vi "Single Command with parameters.vi"(8 "error in (no error)":errorcluster, 9 "Variant (simple type, or Cluster/Array)":variant, 10 "SQL (Single Command)":string, 11 "PQ Connection in":refnum<class "PQ Connection.lvclass">) -> (0 "error out":errorcluster, 1 "First Result with Rows returned":refnum<class "PQ Result.lvclass">, 2 "Number of Rows":i32, 3 "PQ Connection out":refnum<class "PQ Connection.lvclass">)   [LabVIEW 2013, in "PQ Connection.lvclass"]
uses:
  PQ Connection.lvclass
  Result/PQ Result.lvclass
  <userlib>/_OpenG.lib/lvdata/lvdata.llb/Get TDEnum from TD__ogtk.vi
  1. Sources/Lib/Lib.llb/Variant to Header Info__ogtk.vi
  Cluster to Array (recursive).vi
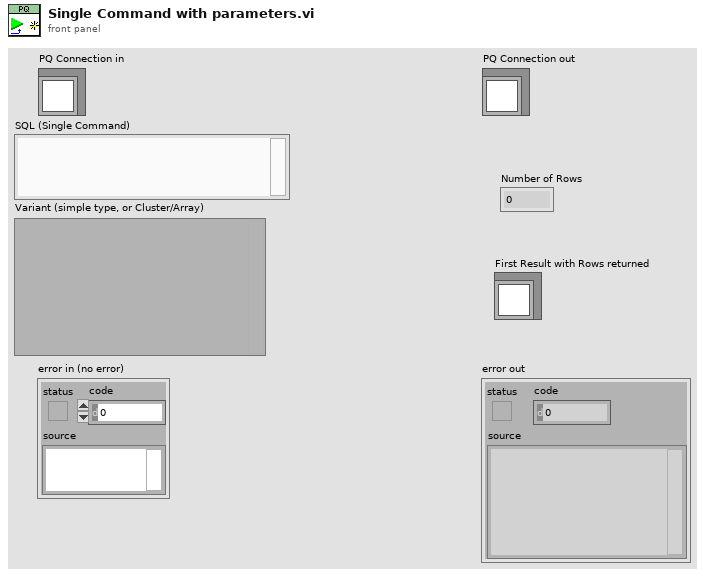
[diagram p1: front panel]
types:
  T1 = enum8{"Invalid Type", "Void", "I8", "I16", "I32", "I64", "U8", "U16", "U32", "U64", "Single Float", "Double Float", "Extended Float", "Single Complex", "Double Complex", "Extended Complex", "Enum U8", "Enum U16", "Enum U32", "Enum U64", "Single Float With Unit", "Double Float With Unit", "Extended Float With Unit", "Single Complex with Unit", "Double Complex with Unit", "Extended Complex with Unit", "Boolean", "String", "Path", "Picture", "Tag", "Array", "Cluster", "Variant", "LV Variant", "Waveform", "Timestamp", "Digital Waveform", "Digital Data", "ExpressData", "Refnum", "External Data", "VI", "Poly VI", "LabVIEW Class Instance", "Fixed Point"}[]
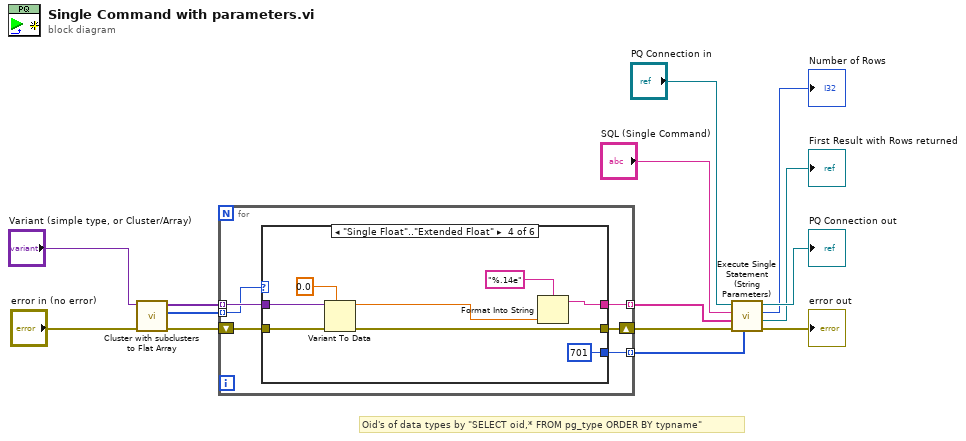
[diagram p0: block diagram]
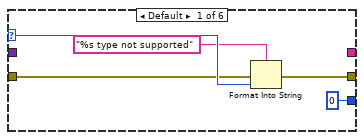
[diagram p2: hidden frame]
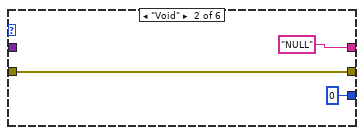
[diagram p3: hidden frame]
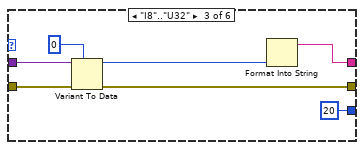
[diagram p4: hidden frame]
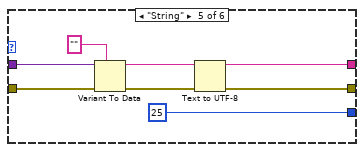
[diagram p5: hidden frame]
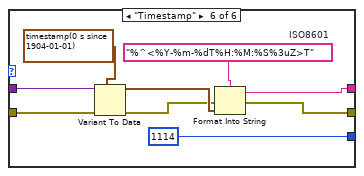
[diagram p6: hidden frame]
diagram:
  # "Oid's of data types by \"SELECT oid,* FROM pg_type ORDER BY typname\""
  n1 = call "Cluster with subclusters to Flat Array.vi"("error in (no error)"="error in (no error)", "Variant"="Variant (simple type, or Cluster/Array)") -> ("error out"=w13:errorcluster, "Types"=w1:T1, "Array of items"=w14:variant[])  [unwired: 7 in]
  n2 = for {
    tunnel: w14 -> [w20] mode=indexing
    tunnel: [w19] -> w7 mode=indexing
    shift-right: [w18] -> w8
    shift-left: w13 -> [w15]
    tunnel: [w17] -> w2 mode=indexing
    tunnel: w1 -> [w16] mode=indexing
    n3 = case shown="\"Single Float\"..\"Extended Float\"" w16 {
      selector: w16 -> [w25 _ _ _ _ _]
      tunnel: w20 -> [_ _ w35 w43 w51 w60]
      tunnel: [_ "NULL" w32 w40 w46 w52] -> w19
      tunnel: w15 -> [w23 w27 w31 w38 w49 w59]
      tunnel: [w22 w27 w30 w37 w44 w53] -> w18
      tunnel: [0 0 20 701 25 1114] -> w17
      frame Default {
        n4 = Format Into String(format string="%s type not supported", error in=w23, w25) -> (error out=w22:errorcluster)  [unwired: 1 in, 1 out]
      }
      frame "Void" {
      }
      frame "I8".."U32" {
        n5 = Variant To Data(error in=w31, type=i64 0, Variant=w35) -> (data=w33:i64, error out=w30:errorcluster)
        n6 = Format Into String(w33) -> (resulting string=w32:string)  [unwired: 3 in, 1 out]
      }
      frame "Single Float".."Extended Float" {
        n7 = Variant To Data(error in=w38, type=0.0, Variant=w43) -> (data=w41:dbl, error out=w37:errorcluster)
        n8 = Format Into String(format string="%.14e", w41) -> (resulting string=w40:string)  [unwired: 2 in, 1 out]
      }
      frame "String" {
        n9 = Variant To Data(error in=w49, type="", Variant=w51) -> (data=w47:string, error out=w45:errorcluster)
        n10 = Text to UTF-8(8:w45, 11:w47) -> (0:w44:errorcluster, 3:w46:string)
      }
      frame "Timestamp" {
        w56 = "%^<%Y-%m-%dT%H:%M:%S%3uZ>T"  # ISO8601
        n11 = Variant To Data(error in=w59, type=timestamp(0 s since 1904-01-01), Variant=w60) -> (data=w55:timestamp, error out=w54:errorcluster)
        n12 = Format Into String(format string=w56, error in=w54, w55) -> (resulting string=w52:string, error out=w53:errorcluster)  [unwired: 1 in]
      }
    }
  }
  n13 = call "Execute Single Statement (String Parameters).vi"("Oids"=w2, "error in (no error)"=w8, "Parameters"=w7, "SQL (Single Command)"="SQL (Single Command)", "PQ Connection in"="PQ Connection in") -> ("error out"=→"error out":errorcluster, "First Result with Rows returned"=→"First Result with Rows returned":refnum<class "PQ Result.lvclass">, "Number of Rows"=→"Number of Rows":i32, "PQ Connection out"=→"PQ Connection out":refnum<class "PQ Connection.lvclass">)  [unwired: 3 in]
